vi "ToAbsolutePath.vi"(11 "relative path":string) -> (3 "absolute path":string)   [LabVIEW 2009]
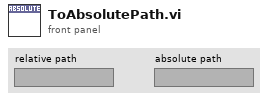
[diagram p1: front panel]
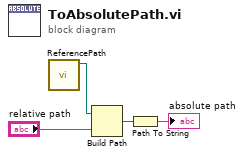
[diagram p0: block diagram]
diagram:
  n1 = call "ReferencePath.vi"() -> ("relative path"=w4:path)  [unwired: 11 in]
  n2 = Build Path(base path=w4, name or relative path="relative path") -> (appended path=w2:path)
  n3 = Path To String(path=w2) -> (string=→"absolute path":string)
